vi "Facade.vi"(0 "Data In":T29 {"Filter"."Stages"."IIR Filter"."Forward Coefficients" format="%.4f"; "Filter"."Stages"."IIR Filter"."Reverse Coefficients" format="%.4f"}, 2 "Display State In":T27, 3 "Container State":T28) -> (6 "Data Out":T29 {"Filter"."Stages"."IIR Filter"."Forward Coefficients" format="%.4f"; "Filter"."Stages"."IIR Filter"."Reverse Coefficients" format="%.4f"}, 7 "Display State Out":T27, 8 "Action":T26)   [LabVIEW 2020, in "Multichannel (Full).xctl"]
uses:
  Multichannel (Full).xctl
  Data.ctl
  Stimulus Channel (Full)/Full Stimulus Channel Data.ctl
  Waveform XCtl/Waveform Data.ctl
  Waveform XCtl/Waveform Enum.ctl
  Waveform VIs/Tone VIs/Tone Params.ctl
  Waveform VIs/Pulse Train VIs/Pulse Train Params.ctl
  Waveform VIs/Pulse Train VIs/Pulse Polarity.ctl
  Waveform VIs/Pulse Train VIs/PT-Continuous State.ctl
  Waveform VIs/Noise VIs/Noise Params.ctl
  Waveform VIs/File VIs/StimFile-Params.ctl
  Waveform VIs/FM Sweep VIs/FM Sweep Params.ctl
  Waveform VIs/Chirp Train VIs/Chirp Train.ctl
  Waveform VIs/Chirp Train VIs/Chirp Train Params.ctl
  Waveform VIs/Complex Tone VIs/CT-Params.ctl
  Waveform VIs/Complex Tone VIs/CT-Phase Enum.ctl
  Waveform VIs/Complex Tone VIs/CT-Runtime Data.ctl
  Waveform VIs/Moving Ripple VIs/Moving Ripple.ctl
  Waveform VIs/Moving Ripple VIs/Moving Ripple.Params.ctl
  Waveform VIs/Moving Ripple VIs/Moving Ripple.Data.ctl
  Advanced Filter XCtl/Filter Data.ctl
  Filter VIs/Filter-Bandwidth Units.ctl
  Burst XCtl/Burst Data.ctl
  Level XCtl/Level Data.ctl
  Level XCtl/Level Units.ctl
  Advanced Options XCtl/Advanced Stimulus Options.ctl
  Modulation VIs/SAM VIs/SAM Params.ctl
  <vilib>/_xctls/Container State.ctl
  State.ctl
  <vilib>/_xctls/Action.ctl
  Stimulus Channel (Full)/Stimulus Channel (Full).xctl
  <vilib>/_xctls/XControlSupport.lvlib
  Level XCtl/Level XCtl.xctl
  Waveform XCtl/Waveform XCtl.xctl
  Burst XCtl/Burst Control.xctl
  Advanced Filter XCtl/Advanced Filter XCtl.xctl
  Advanced Options XCtl/Advanced Stimulus Options.xctl
panel:
  in  "Channel list":i32(listbox)
  in  "Stimulus Params":T25(xcontrol)
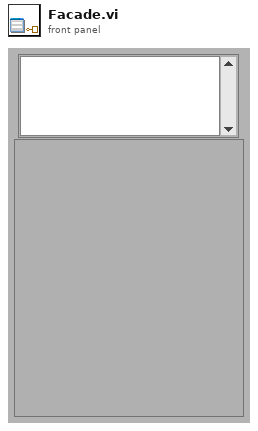
[diagram p1: front panel]
types:
  T1 = typedef "Waveform XCtl.xctl/Waveform Data.ctl" = cluster{"Type":T2, "Tone":T3, "Pulse Train":T4, "Noise":T7, "File":T8, "FMSweep":T9, "Chirp Train":T10, "Complex Tone":cluster{"Params":T12, "Data":T14}, "Moving Ripple":T15}
  T2 = typedef "Waveform Enum.ctl" = enum16{"OFF", "Tone", "Noise", "Pulse Train", "File", "FM Sweep", "Chirp Train", "Complex Tone", "FM Tone", "Moving Ripple"}
  T3 = typedef "Tone Params.ctl" = cluster{"Frequency (kHz)":dbl, "Last Freq":dbl, "Last Phase":dbl}
  T4 = typedef "Pulse Train Params.ctl" = cluster{"Pulse width (us)":dbl, "Pulse rate (Hz)":dbl, "Gap (ms)":dbl, "Polarity":T5, "PT State":T6, "Asynch":bool}
  T5 = typedef "Pulse Polarity.ctl" = enum16{"POS", "NEG", "POS-NEG", "NEG-POS"}
  T6 = typedef "PT-Continuous State.ctl" = cluster{"Template":dbl[], "Nperiod":i32, "Index":i32, "Pulse Rate (Hz)":dbl, "Phase (cycles)":dbl, "Noff":i32}
  T7 = typedef "Noise Params.ctl" = cluster{"InvFilt":bool, "Noise":dbl[], "CurPt":i32, "Aweight":bool, "Seed":i32, "afile":path}
  T8 = typedef "StimFile-Params.ctl" = cluster{"Filename":path, "Signal":dbl[], "Channel":i32, "stream":bool, "offset":i32, "nreps":i32, "loops":i32, "Randomize":bool, "order":i32[], "Seed":i32, "Tokens":i32}
  T9 = typedef "FM Sweep Params.ctl" = cluster{"Rate (oct/s)":dbl, "Fmin (Hz)":dbl, "Fmax (Hz)":dbl, "Ramp (ms)":dbl, "Linear":bool}
  T10 = typedef "Chirp Train.ctl" = cluster{"Params":T11, "Data":cluster{"WF":dbl[]}}
  T11 = typedef "Chirp Train Params.ctl" = cluster{"Fmin (kHz)":dbl, "Fmax (kHz)":dbl, "Compensate":bool, "Duration (ms)":dbl}
  T12 = typedef "CT-Params.ctl" = cluster{"F0 (Hz)":dbl, "Band":cluster{"Flow (Hz)":dbl, "Fhigh (Hz)":dbl}, "Phase":T13, "Min F0 (Hz)":dbl, "Max F0 (Hz)":dbl, "ContinRandPhase":bool, "Max peak factor":dbl, "Max mod depth":dbl, "MinHarmNum":i32, "MaxHarmNum":i32, "Level Mode":enum16{"per component", "overall rms"}, "% jitter":dbl}
  T13 = typedef "CT-Phase Enum.ctl" = enum16{"Cosine", "Random", "Alternating"}
  T14 = typedef "CT-Runtime Data.ctl" = cluster{"Ncomp":i32, "MinHarm":i32, "Phase":dbl[], "Amplitude":dbl[], "Npts/frame":i32, "Last F0":dbl, "Fmin":dbl, "Fmax":dbl, "Lslope":dbl, "randphase":bool, "overall rms":bool, "fmult":dbl[], "jittered":bool}
  T15 = typedef "Moving Ripple.ctl" = cluster{"Params":T16, "Data":T17}
  T16 = typedef "Moving Ripple.Params.ctl" = cluster{"Fmin":dbl, "Fmax":dbl, "Density":dbl, "Velocity":dbl, "Depth":dbl, "Phase":dbl, "Comp/oct":i32}
  T17 = typedef "Moving Ripple.Data.ctl" = cluster{"Freq":dbl[], "A":dbl[], "phase":dbl[], "Phase":dbl}
  T18 = typedef "Advanced Filter XCtl.xctl/Filter Data.ctl" = cluster{"Type":enum16{"Lowpass", "Highpass", "Bandpass", "Bandstop", "OFF"}, "CF (kHz)":dbl, "BW (kHz)":dbl, "Cascade":bool, "Quadrature":bool, "Scale Factor":dbl, "Stages":cluster{"IIR Filter":cluster{"filter structure":enum32{"IIR 2nd Order", "IIR 4th Order"}, "Reverse Coefficients":dbl[], "Forward Coefficients":dbl[]}, "State":dbl[]}[], "Class":enum16{"Elliptic", "Butterworth"}, "Order":i32, "BWUnits":T19}
  T19 = typedef "Filter-Bandwidth Units.ctl" = enum16{"Linear", "Octaves", "Min-Max"}
  T20 = typedef "Burst Control.xctl/Burst Data.ctl" = cluster{"Active":bool, "Delay (ms)":dbl, "Duration (ms)":dbl, "Ramp (ms)":dbl, "Rate (Hz)":dbl, "Trepeat (ms)":dbl, "Repeat":bool}
  T21 = typedef "Level XCtl.xctl/Level Data.ctl" = cluster{"Level":dbl, "Units":T22, "Max":dbl, "Multiplier":dbl, "Cal File":path, "Cal":cluster{"Freq (Hz)":dbl[], "Mag (dB SPL)":dbl[], "Phase (deg)":dbl[]}}
  T22 = typedef "Level Units.ctl" = enum16{"dB atten", "dB SPL", "dB re 1 Vrms", "dB V/Hz½", "mW", "dB HL", "Volts", "dB mW"}
  T23 = typedef "Advanced Stimulus Options.xctl/Advanced Stimulus Options.ctl" = cluster{"Rep Mask":string, "AltPol":bool, "Var":string, "Expr":string, "Persist":bool}
  T24 = typedef "SAM Params.ctl" = cluster{"Active":bool, "Frequency (Hz)":dbl, "Depth":dbl, "Init Phase (cycles)":dbl, "phase (degrees)":dbl, "Asynch":bool}
  T25 = cluster{"Waveform":T1, "Filter":T18, "Burst":T20, "Level":T21, "Name":string, "Advanced":T23, "SAM":T24}
  T26 = typedef "XControlSupport.lvlib/Action.ctl" = cluster{"Data Changed?":bool, "State Changed?":bool, "Action Name":string}
  T27 = typedef "Multichannel (Full).xctl/State.ctl" = cluster{"names":string[], "Reinit?":bool, "Advanced?":bool, "Validate?":bool, "Show persist":bool}
  T28 = typedef "XControlSupport.lvlib/Container State.ctl" = cluster{"Indicator?":bool, "Run Mode?":bool, " Refnum":refnum<vi>}
  T29 = typedef "Multichannel (Full).xctl/Data.ctl" = T30[]
  T30 = typedef "Stimulus Channel (Full).xctl/Full Stimulus Channel Data.ctl" = cluster{"Waveform":T1, "Filter":T18, "Burst":T20, "Level":T21, "Name":string, "Advanced":T23, "SAM":T24}
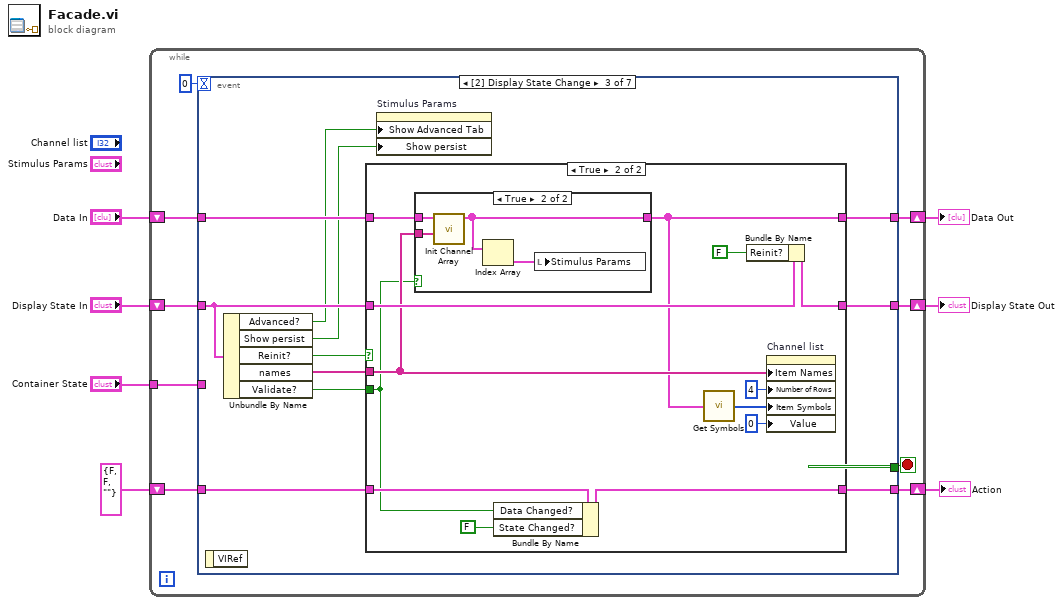
[diagram p0: block diagram]
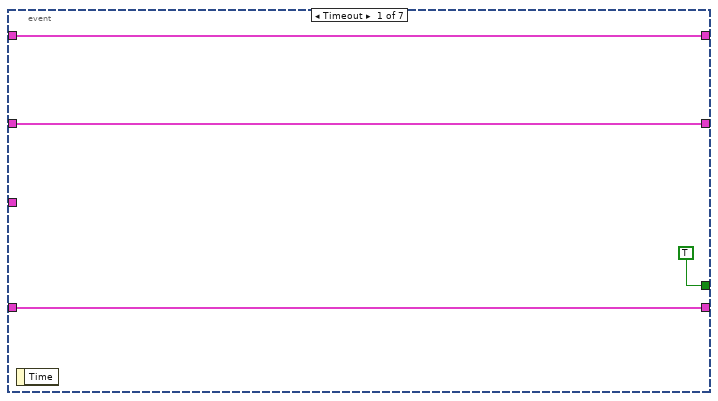
[diagram p2: hidden frame]
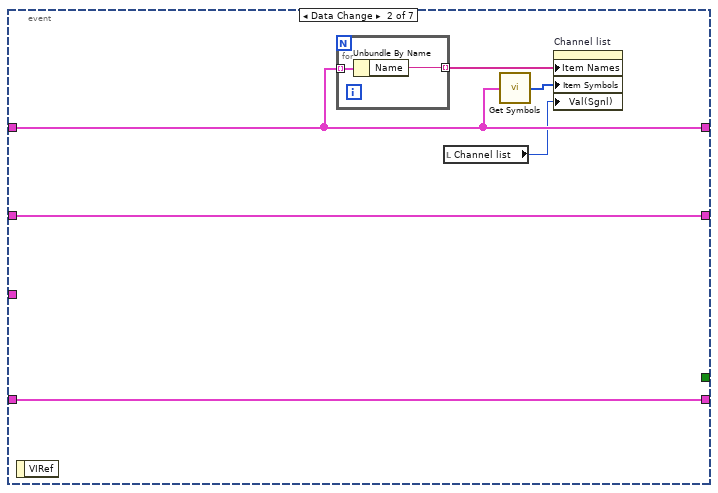
[diagram p3: hidden frame]
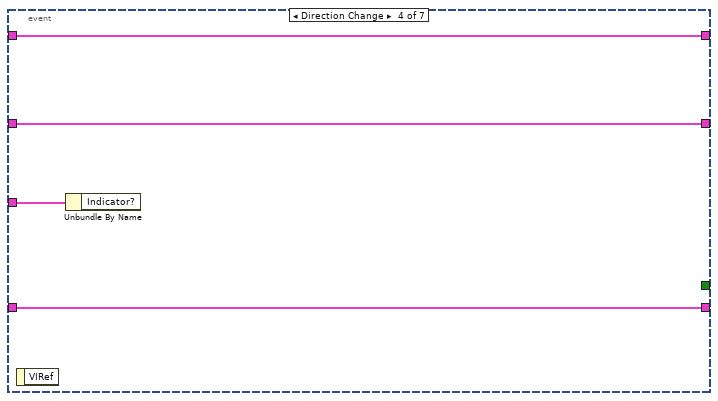
[diagram p6: hidden frame]
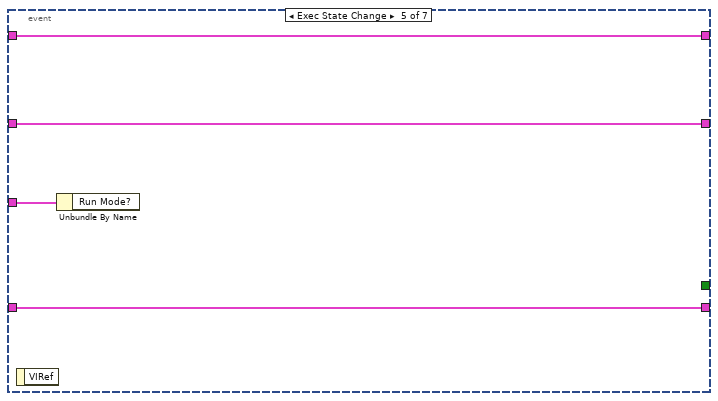
[diagram p7: hidden frame]
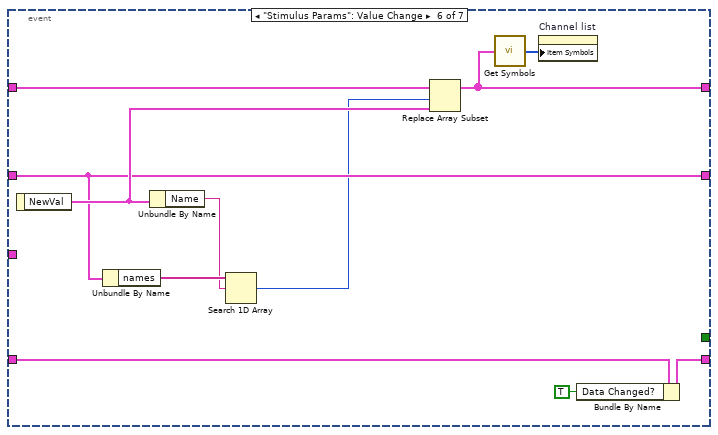
[diagram p8: hidden frame]
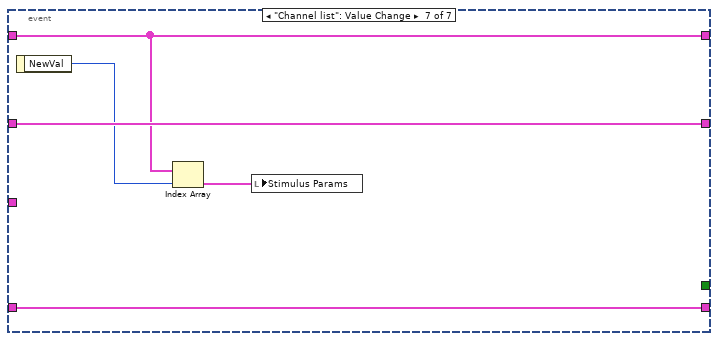
[diagram p9: hidden frame]
diagram:
  n1 = while {
    shift-right: [w15] -> w4
    shift-left: "Display State In" -> [w16]
    tunnel: "Container State" -> [w12]
    shift-right: [w10] -> w7
    shift-left: "Data In" -> [w11]
    shift-right: [w8] -> w2
    shift-left: T26 {"Data Changed?"=FALSE, "State Changed?"=FALSE, "Action Name"=""} ("Action") -> [w9]
    stop <- w14 stop-if-true
    n2 = event shown="[2] Display State Change" {
      selector: _ -> [_ _ _ _ _ _ _]
      dyn-events: _ -> [_ _ _ _ _ _ _]
      timeout: 0 -> [_ _ _ _ _ _ _]
      tunnel: w16 -> [w18 w26 w36 w63 w67 w75 w84]
      tunnel: [w18 w26 w35 w63 w67 w75 w84] -> w15
      tunnel: [TRUE _ _ _ _ _ _] -> w14
      tunnel: w12 -> [_ _ _ w64 w68 _ _]
      tunnel: w11 -> [w17 w24 w38 w62 w66 w79 w83]
      tunnel: [w17 w24 w37 w62 w66 w71 w83] -> w10
      tunnel: [w19 w25 w33 w61 w65 w76 w81] -> w8
      tunnel: w9 -> [w19 w25 w34 w61 w65 w77 w81]
      event Timeout {
        n3 = event-data() -> ()  [unwired: 1 in, 1 out]
      }
      event Data Change {
        n4 = event-data() -> ()  [unwired: 1 in, 1 out]
        n5 = for {
          tunnel: w24 -> [w28] mode=indexing
          tunnel: [w27] -> w22 mode=indexing
          n6 = Unbundle By Name(w28) -> ("Name"=w27:string)
        }
        n7 = local read "Channel list"() -> (w21:i32)
        n8 = call "Get Symbols.vi"("Multichannel"=w24) -> ("Symbols"=w23:i32[])
        n9 = property on="Channel list" class="LstBox (strict)"("Item Names"=w22, "Item Symbols"=w23, "Val(Sgnl)"=w21) -> ()  [unwired: 2 in, 2 out]
      }
      event Display State Change {
        n10 = event-data() -> ()  [unwired: 1 in, 1 out]
        n11 = Unbundle By Name(w36) -> ("Advanced?"=w31:bool, "Show persist"=w29:bool, "Reinit?"=w39:bool, "names"=w32:string[], "Validate?"=w30:bool)
        n12 = case shown="True" w39 {
          tunnel: w38 -> [w42 w50]
          tunnel: [w42 w43] -> w37
          tunnel: w36 -> [w41 w53]
          tunnel: [w41 w52] -> w35
          tunnel: w34 -> [w40 w55]
          tunnel: [w40 w54] -> w33
          tunnel: w32 -> [_ w48]
          tunnel: w30 -> [_ w44]
          frame False {
          }
          frame True {
            n13 = case shown="True" w44 {
              tunnel: w50 -> [w56 w60]
              tunnel: w48 -> [_ w59]
              tunnel: [w56 w57] -> w43
              frame False {
              }
              frame True {
                n14 = call "Init Channel Array.vi"("Names"=w59, "Data In"=w60) -> ("Data out"=w57:T29)  [unwired: 9 in]
                n15 = Index Array(array=w57) -> (element=w58:T30)  [unwired: 1 in]
                n16 = local write "Stimulus Params"(w58) -> ()
              }
            }
            n17 = Bundle By Name(cluster=w55, "Data Changed?"=w44, "State Changed?"=FALSE ("Data Changed?")) -> (w54:T26)
            n18 = call "Get Symbols.vi"("Multichannel"=w43) -> ("Symbols"=w47:i32[])
            n19 = Bundle By Name(cluster=w53, "Reinit?"=FALSE) -> (w52:T27)
            n20 = property on="Channel list" class="LstBox (strict)"("Item Names"=w48, "Number of Rows"=u32 4, "Item Symbols"=w47, "Value"=0 ("Channel list")) -> ()  [unwired: 2 in, 2 out]
          }
        }
        n21 = property on="Stimulus Params" class="Stimulus Channel (Full) (strict"("Show Advanced Tab"=w31, "Show persist"=w29) -> ()  [unwired: 2 in, 2 out]
      }
      event Direction Change {
        n22 = event-data() -> ()  [unwired: 1 in, 1 out]
        n23 = Unbundle By Name(w64) -> ()  [unwired: 1 out]
      }
      event Exec State Change {
        n24 = event-data() -> ()  [unwired: 1 in, 1 out]
        n25 = Unbundle By Name(w68) -> ()  [unwired: 1 out]
      }
      event "Stimulus Params": Value Change {
        n26 = event-data() -> ("NewVal"=w78:T25)  [unwired: 1 in]
        n27 = Unbundle By Name(w75) -> ("names"=w73:string[])
        n28 = Unbundle By Name(w78) -> ("Name"=w72:string)
        n29 = Search 1D Array(1D array=w73, element=w72) -> (index of element=w69:i32)  [unwired: 1 in]
        n30 = Replace Array Subset(array=w79, new element=w78, index=w69) -> (w71:T29)
        n31 = call "Get Symbols.vi"("Multichannel"=w71) -> ("Symbols"=w70:i32[])
        n32 = property on="Channel list" class="LstBox (strict)"("Item Symbols"=w70) -> ()  [unwired: 2 in, 2 out]
        n33 = Bundle By Name(cluster=w77, "Data Changed?"=TRUE) -> (w76:T26)
      }
      event "Channel list": Value Change {
        n34 = event-data() -> ("NewVal"=w82:i32)  [unwired: 1 in]
        n35 = Index Array(array=w83, index=w82) -> (element=w80:T30)
        n36 = local write "Stimulus Params"(w80) -> ()
      }
    }
  }
  "Display State Out" <- w4
  "Data Out" <- w7
  "Action" <- w2
